vi "Agilent VNA Set Learn String.vi"(7 "Agilent VNA":T1, 8 "error in (no error)":errorcluster, 10 "Learn String":string, 11 "VISA Resource Name":refnum<visa-resource-name>) -> (0 "error out":errorcluster {"code" format="%.0x"}, 3 "dup VISA Resource Name":refnum<visa-resource-name>)   [LabVIEW 2011]
uses:
  TypeDefs/Agilent VNA Instrument Info.ctl
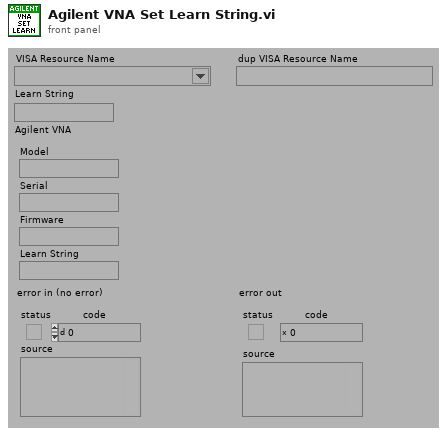
[diagram p1: front panel]
types:
  T1 = typedef "Agilent VNA Instrument Info.ctl" = cluster{"Model":string, "Serial":string, "Firmware":string, "Learn String":string}
  T2 = typedef "Agilent VNA Model.ctl" = enum16{"Not Supported", "8510X", "8719X", "8720X", "8722X", "8753X", "ENA", "PNA", "Field Fox"}
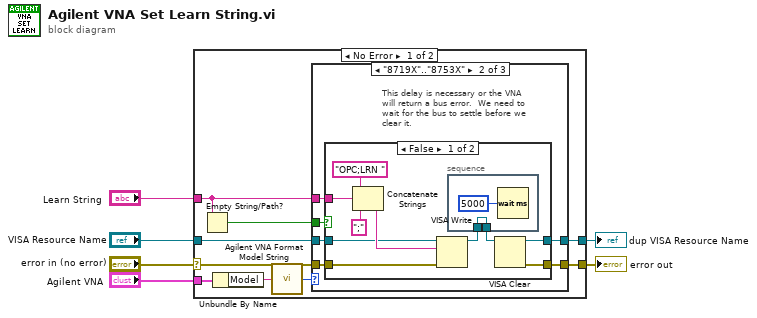
[diagram p0: block diagram]
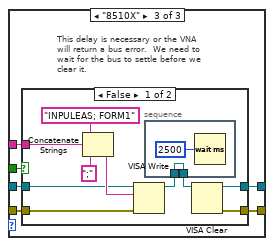
[diagram p4: hidden frame]
diagram:
  n1 = case shown="No Error" "error in (no error)" {
    selector: "error in (no error)" -> [w7 w58]
    tunnel: [w15 w58] -> w6
    tunnel: "Learn String" -> [w13 _]
    tunnel: "VISA Resource Name" -> [w12 w59]
    tunnel: [w11 w59] -> w3
    tunnel: "Agilent VNA" -> [w9 _]
    frame No Error {
      n2 = Empty String/Path?(string/path=w13) -> (empty?=w14:bool)
      n3 = Unbundle By Name(w9) -> ("Model"=w8:string)
      n4 = call "Agilent VNA Format Model String.vi"("Model"=w8) -> ("Model"=w10:T2)
      n5 = case shown="\"8719X\"..\"8753X\"" w10 {
        tunnel: [w16 w23 w43] -> w15
        tunnel: w7 -> [w16 w22 w42]
        tunnel: w14 -> [_ w21 w41]
        tunnel: w13 -> [_ w20 w40]
        tunnel: w12 -> [w17 w19 w39]
        tunnel: [w17 w18 w38] -> w11
        frame "Not Supported", "ENA".."Field Fox" {
        }
        frame "8719X".."8753X" {
          # "This delay is necessary or the VNA\nwill return a bus error.  We need to\nwait for the bus to settle before we\nclear it."
          n6 = case shown="False" w21 {
            tunnel: [w27 w37] -> w23
            tunnel: w22 -> [w30 w37]
            tunnel: w20 -> [w29 _]
            tunnel: w19 -> [w28 w36]
            tunnel: [w26 w36] -> w18
            frame False {
              n7 = Concatenate Strings("OPC;LRN ", w29, ";") -> (w31:string)
              n8 = VISA Write(VISA resource name=w28, write buffer=w31, error in (no error)=w30) -> (VISA resource name out=w25:refnum<visa-resource-name>)  [unwired: 2 out]
              n9 = stacked-sequence {
                tunnel: w25 -> [w34]
                tunnel: [w34] -> w24
                frame #0 {
                  n10 = Wait (ms)(milliseconds to wait=u32 5000) -> ()  [unwired: 1 out]
                }
              }
              n11 = VISA Clear(VISA resource name=w24) -> (VISA resource name out=w26:refnum<visa-resource-name>, error out=w27:errorcluster)  [unwired: 1 in]
            }
            frame True {
            }
          }
        }
        frame "8510X" {
          # "This delay is necessary or the VNA\nwill return a bus error.  We need to\nwait for the bus to settle before we\nclear it."
          n12 = case shown="False" w41 {
            tunnel: [w47 w57] -> w43
            tunnel: w42 -> [w50 w57]
            tunnel: w40 -> [w49 _]
            tunnel: w39 -> [w48 w56]
            tunnel: [w46 w56] -> w38
            frame False {
              n13 = Concatenate Strings("INPULEAS; FORM1", w49, ";") -> (w51:string)
              n14 = VISA Write(VISA resource name=w48, write buffer=w51, error in (no error)=w50) -> (VISA resource name out=w45:refnum<visa-resource-name>)  [unwired: 2 out]
              n15 = stacked-sequence {
                tunnel: w45 -> [w54]
                tunnel: [w54] -> w44
                frame #0 {
                  n16 = Wait (ms)(milliseconds to wait=u32 2500) -> ()  [unwired: 1 out]
                }
              }
              n17 = VISA Clear(VISA resource name=w44) -> (VISA resource name out=w46:refnum<visa-resource-name>, error out=w47:errorcluster)  [unwired: 1 in]
            }
            frame True {
            }
          }
        }
      }
    }
    frame Error {
    }
  }
  "error out" <- w6
  "dup VISA Resource Name" <- w3
